vi "Write Text Labels[].vi"(8 "error in (no error)":errorcluster, 10 "TextLbls[]":string[](array[string]), 11 "NumericWithScale.lvclass in":refnum<class "NumericWithScale.lvclass">) -> (0 "error out":errorcluster, 3 "NumericWithScale.lvclass out":refnum<class "NumericWithScale.lvclass">)   [LabVIEW 2015, in "NumericWithScale.lvclass"]
uses:
  NumericWithScale.lvclass
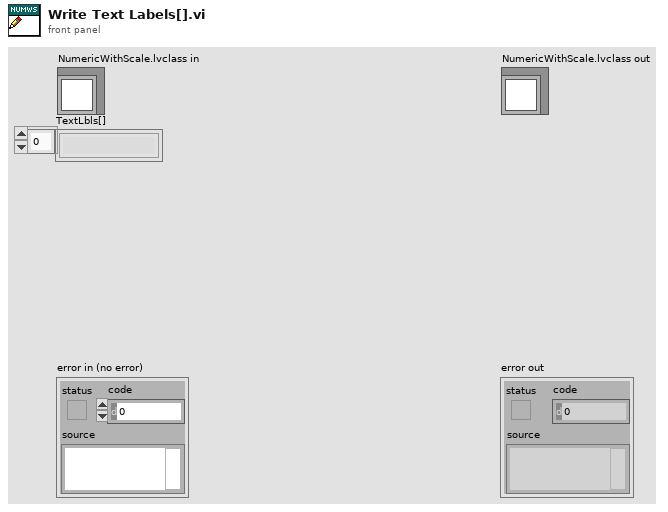
[diagram p1: front panel]
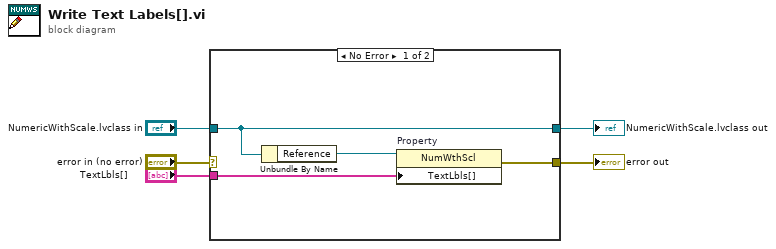
[diagram p0: block diagram]
diagram:
  n1 = case shown="No Error" "error in (no error)" {
    selector: "error in (no error)" -> [_ w11]
    tunnel: [w9 w11] -> w4
    tunnel: [w7 w10] -> w2
    tunnel: "NumericWithScale.lvclass in" -> [w7 w10]
    tunnel: "TextLbls[]" -> [w8 _]
    frame No Error {
      n2 = Unbundle By Name(w7) -> ("Reference"=w6:refnum<vi>)
      n3 = property on="Property" class="NumWthScl"(reference=w6, "TextLbls[]"=w8) -> (error out=w9:errorcluster)  [unwired: 1 in, 1 out]
    }
    frame Error {
    }
  }
  "error out" <- w4
  "NumericWithScale.lvclass out" <- w2
